vi "pressure formulas (SubVI).vi"(0 "Numeric 18":u16, 1 "Numeric 16":u16, 2 "Numeric in":u16, 3 "Numeric 14":u16, 4 "Numeric 4":u16, 5 "Numeric 12":u16, 6 "Numeric 6":u16, 7 "Numeric 10":u16, 8 "Numeric 20":u16, 9 "Numeric 8":u16) -> (10 "Numeric 5":dbl, 11 "Numeric 9":dbl, 12 "Numeric 3":dbl, 13 "Numeric 11":dbl, 14 "Numeric 19":dbl, 15 "Numeric out":dbl, 16 "Numeric 7":dbl, 17 "Numeric 17":dbl, 18 "Numeric 15":dbl, 19 "Numeric 13":dbl)   [LabVIEW 2016]
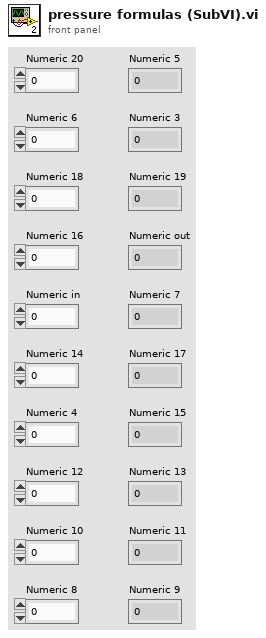
[diagram p1: front panel]
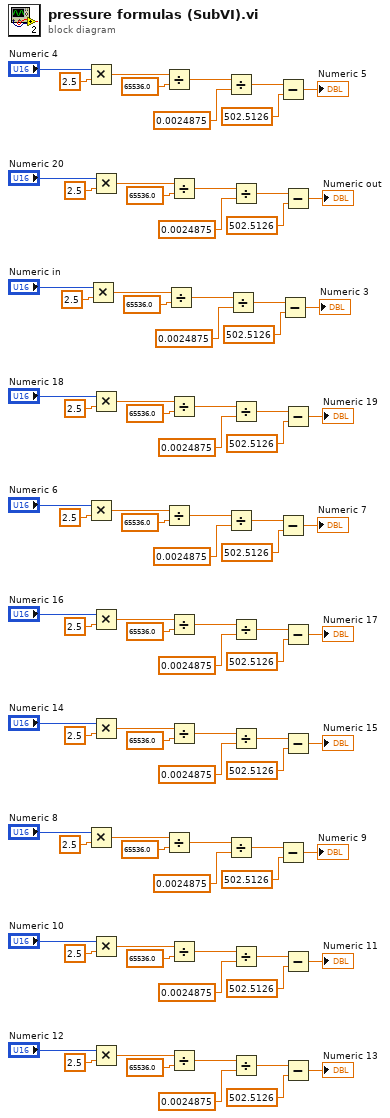
[diagram p0: block diagram]
diagram:
  n1 = Multiply(x="Numeric 4", y=2.5) -> (x*y=w84:dbl)
  n2 = Multiply(x="Numeric 6", y=2.5) -> (x*y=w79:dbl)
  n3 = Multiply(x="Numeric 8", y=2.5) -> (x*y=w74:dbl)
  n4 = Multiply(x="Numeric in", y=2.5) -> (x*y=w89:dbl)
  n5 = Multiply(x="Numeric 20", y=2.5) -> (x*y=w39:dbl)
  n6 = Multiply(x="Numeric 18", y=2.5) -> (x*y=w43:dbl)
  n7 = Multiply(x="Numeric 16", y=2.5) -> (x*y=w51:dbl)
  n8 = Multiply(x="Numeric 14", y=2.5) -> (x*y=w57:dbl)
  n9 = Multiply(x="Numeric 10", y=2.5) -> (x*y=w69:dbl)
  n10 = Multiply(x="Numeric 12", y=2.5) -> (x*y=w64:dbl)
  n11 = Divide(x=w84, y=65536.0) -> (x/y=w82:dbl)
  n12 = Divide(x=w79, y=65536.0) -> (x/y=w77:dbl)
  n13 = Divide(x=w74, y=65536.0) -> (x/y=w72:dbl)
  n14 = Divide(x=w89, y=65536.0) -> (x/y=w87:dbl)
  n15 = Divide(x=w39, y=65536.0) -> (x/y=w41:dbl)
  n16 = Divide(x=w43, y=65536.0) -> (x/y=w45:dbl)
  n17 = Divide(x=w51, y=65536.0) -> (x/y=w53:dbl)
  n18 = Divide(x=w57, y=65536.0) -> (x/y=w58:dbl)
  n19 = Divide(x=w69, y=65536.0) -> (x/y=w67:dbl)
  n20 = Divide(x=w64, y=65536.0) -> (x/y=w62:dbl)
  n21 = Divide(x=w82, y=0.0024875) -> (x/y=w85:dbl)
  n22 = Divide(x=w77, y=0.0024875) -> (x/y=w80:dbl)
  n23 = Divide(x=w72, y=0.0024875) -> (x/y=w75:dbl)
  n24 = Divide(x=w87, y=0.0024875) -> (x/y=w90:dbl)
  n25 = Divide(x=w41, y=0.0024875) -> (x/y=w47:dbl)
  n26 = Divide(x=w45, y=0.0024875) -> (x/y=w50:dbl)
  n27 = Divide(x=w53, y=0.0024875) -> (x/y=w55:dbl)
  n28 = Divide(x=w58, y=0.0024875) -> (x/y=w60:dbl)
  n29 = Divide(x=w67, y=0.0024875) -> (x/y=w70:dbl)
  n30 = Divide(x=w62, y=0.0024875) -> (x/y=w65:dbl)
  n31 = Subtract(x=w85, y=502.5126) -> (x-y=→"Numeric 5":dbl)
  n32 = Subtract(x=w80, y=502.5126) -> (x-y=→"Numeric 7":dbl)
  n33 = Subtract(x=w75, y=502.5126) -> (x-y=→"Numeric 9":dbl)
  n34 = Subtract(x=w90, y=502.5126) -> (x-y=→"Numeric 3":dbl)
  n35 = Subtract(x=w47, y=502.5126) -> (x-y=→"Numeric out":dbl)
  n36 = Subtract(x=w50, y=502.5126) -> (x-y=→"Numeric 19":dbl)
  n37 = Subtract(x=w55, y=502.5126) -> (x-y=→"Numeric 17":dbl)
  n38 = Subtract(x=w60, y=502.5126) -> (x-y=→"Numeric 15":dbl)
  n39 = Subtract(x=w70, y=502.5126) -> (x-y=→"Numeric 11":dbl)
  n40 = Subtract(x=w65, y=502.5126) -> (x-y=→"Numeric 13":dbl)
